vi "set_icon.vi"(8 "error in (no error)":errorcluster, 10 "Icon File Path":path=path "C:/myVIs/NotifyIcon/Icons/ni.ico", 11 "BalloonNotifier in":refnum<class "BalloonNotifier.lvclass">) -> (0 "error out":errorcluster, 3 "BalloonNotifier out":refnum<class "BalloonNotifier.lvclass">)   [LabVIEW 2017, in "BalloonNotifier.lvclass"]
uses:
  BalloonNotifier.lvclass
  System.Windows.Forms
  System.Drawing
  BalloonNotifier.lvclass/BalloonNotifier.ctl
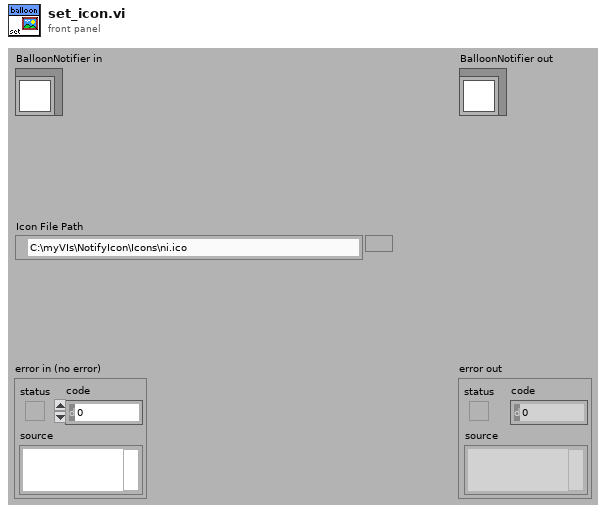
[diagram p1: front panel]
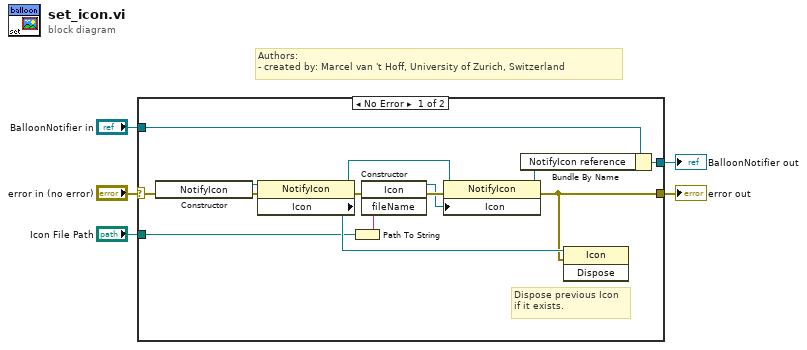
[diagram p0: block diagram]
diagram:
  # "Authors: \n- created by: Marcel van 't Hoff, University of Zurich, Switzerland"
  n1 = case shown="No Error" "error in (no error)" {
    selector: "error in (no error)" -> [w8 w21]
    tunnel: [w12 w21] -> w4
    tunnel: [w9 w20] -> w2
    tunnel: "BalloonNotifier in" -> [w10 w20]
    tunnel: "Icon File Path" -> [w13 _]
    frame No Error {
      # "Dispose previous Icon\nif it exists."
      n2 = constructor class="NotifyIcon"(error in=w8) -> (reference out=w6:refnum<k24>, error out=w7:errorcluster)  [unwired: 2 in, 1 out]
      n3 = property class="NotifyIcon"(reference=w6, error in=w7) -> (reference out=w17:refnum<k24>, error out=w18:errorcluster, "Icon"=w19:refnum<k24>)
      n4 = Path To String(path=w13) -> (string=w14:string)
      n5 = constructor class="Icon"(error in=w18, "fileName"=w14) -> (reference out=w15:refnum<k24>, error out=w16:errorcluster)  [unwired: 2 in, 2 out]
      n6 = property class="NotifyIcon"(reference=w17, error in=w16, "Icon"=w15) -> (reference out=w11:refnum<k24>, error out=w12:errorcluster)
      n7 = Bundle By Name(cluster=w10, "NotifyIcon reference"=w11) -> (w9:refnum<class "BalloonNotifier.lvclass">)
      n8 = invoke class="Icon" method="Dispose"(reference=w19, error in=w12) -> ()  [unwired: 1 in, 3 out]
    }
    frame Error {
    }
  }
  "error out" <- w4
  "BalloonNotifier out" <- w2
